vi "Write AI_AO_ALRState.vi"(0 "OPC UA server refnum in":T4, 1 "AI":T2, 2 "AI tags":string[](array[string]), 3 "AO":dbl[](array[numeric]), 4 "AO tags":string[](array[string]), 5 "error in (no error)":errorcluster, 6 "OPC UA AI list":string[](array[string]), 7 "ALR_State":T1, 9 "ALR tags":string[](array[string])) -> (14 "OPC UA server refnum out":T4, 19 "error out":errorcluster)   [LabVIEW 2019, in "OPC addons.lvlib"]
uses:
  OPC addons.lvlib
  <vilib>/OPCUA/controls/OPC UA Server Refnum.ctl
  Inputs/Ctl/AI short.ctl
  Inputs/Ctl/Parameter State.ctl
  Alarms/Ctl/ALRs_State.ctl
  <vilib>/OPCUA/controls/Write Status.ctl
  <vilib>/OPCUA/server/Write Variant.vi
  <vilib>/OPCUA/NI OPC UA Server.lvlib
  Alarms/Alarms.lvlib
  Inputs/Inputs.lvlib
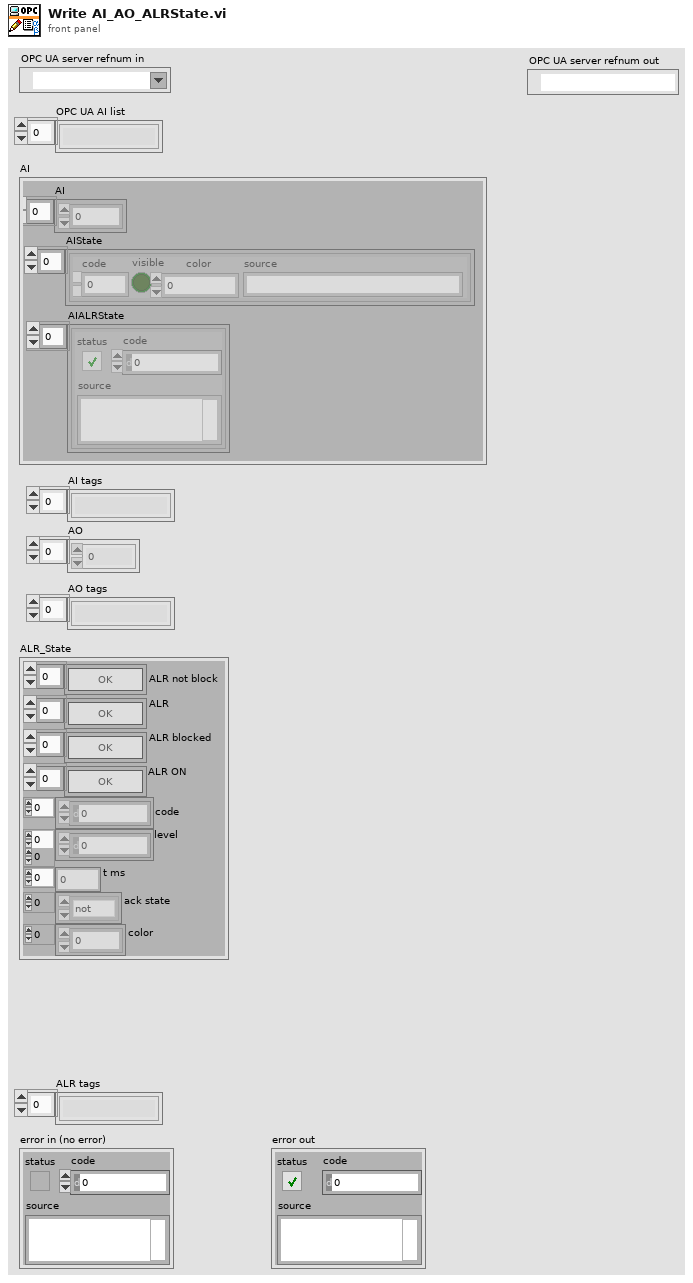
[diagram p1: front panel]
types:
  T1 = typedef "Alarms.lvlib/ALRs_State.ctl" = cluster{"ALR not block":bool[], "ALR":bool[], "ALR blocked":bool[], "ALR ON":bool[], "code":i32[], "level":i32[][], "t ms":u32[], "ack state":enum32{"not", "tripped", "reset", "ack"}[], "color":u32[]}
  T2 = typedef "Inputs.lvlib/AI short.ctl" = cluster{"AI":dbl[], "AIState":T3[], "AIALRState":errorcluster[]}
  T3 = typedef "Inputs.lvlib/Parameter State.ctl" = cluster{"code":i32, "visible":bool, "color":u32, "source":string}
  T4 = typedef "OPC UA Server Refnum.ctl" = refnum<k21>
  T5 = typedef "Write Status.ctl" = u32
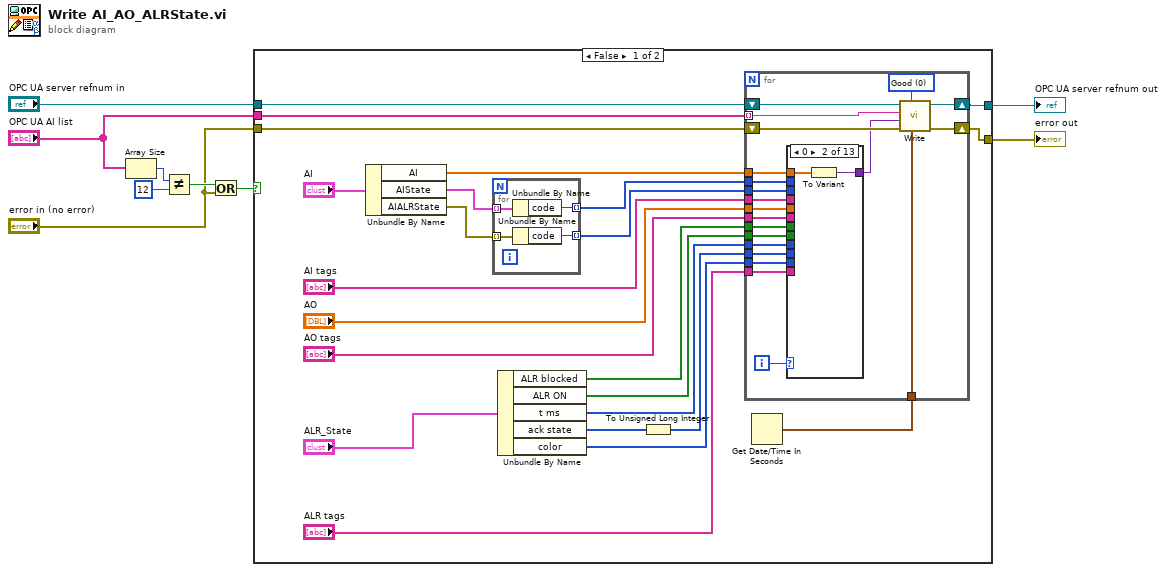
[diagram p0: block diagram]
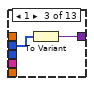
[diagram p3: hidden frame]
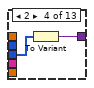
[diagram p4: hidden frame]
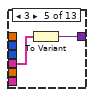
[diagram p5: hidden frame]
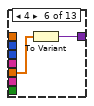
[diagram p6: hidden frame]
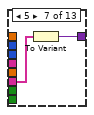
[diagram p7: hidden frame]
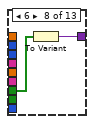
[diagram p8: hidden frame]
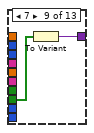
[diagram p9: hidden frame]
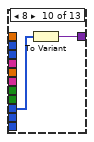
[diagram p10: hidden frame]
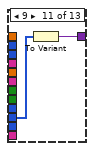
[diagram p11: hidden frame]
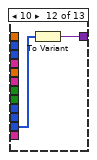
[diagram p12: hidden frame]
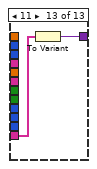
[diagram p13: hidden frame]
diagram:
  n1 = Array Size(array="OPC UA AI list") -> (size(s)=w5:i32)
  n2 = Not Equal?(x=w5, y=12) -> (x != y?=w3:bool)
  n3 = Or(x=w3, y="error in (no error)") -> (x .or. y?=w1:bool)
  n4 = case shown="False" w1 {
    tunnel: "OPC UA server refnum in" -> [w26 w83]
    tunnel: [w25 w83] -> w8
    tunnel: [w24 w82] -> w7
    tunnel: "OPC UA AI list" -> [w23 _]
    tunnel: "error in (no error)" -> [w22 w82]
    frame False {
      n5 = Unbundle By Name("AI") -> ("AI"=w30:dbl[], "AIState"=w31:T3[], "AIALRState"=w32:errorcluster[])
      n6 = for {
        tunnel: w31 -> [w81] mode=indexing
        tunnel: [w80] -> w21 mode=indexing
        tunnel: w32 -> [w79] mode=indexing
        tunnel: [w78] -> w20 mode=indexing
        n7 = Unbundle By Name(w81) -> ("code"=w80:i32)
        n8 = Unbundle By Name(w79) -> ("code"=w78:i32)
      }
      n9 = Unbundle By Name("ALR_State") -> ("ALR blocked"=w17:bool[], "ALR ON"=w18:bool[], "t ms"=w14:u32[], "ack state"=w13:enum32{"not", "tripped", "reset", "ack"}[], "color"=w11:u32[])
      n10 = To Unsigned Long Integer(number=w13) -> (unsigned 32bit integer=w12:u32[])
      n11 = Get Date/Time In Seconds() -> (seconds since 1Jan1904=w28:timestamp)
      n12 = for {
        tunnel: w28 -> [w39]
        tunnel: w30 -> [w53]
        tunnel: w21 -> [w51]
        tunnel: w23 -> [w37] mode=indexing
        tunnel: w20 -> [w50]
        tunnel: "AI tags" -> [w49]
        tunnel: "AO" -> [w48]
        tunnel: "AO tags" -> [w47]
        tunnel: w17 -> [w46]
        tunnel: w18 -> [w45]
        tunnel: w14 -> [w44]
        tunnel: w12 -> [w43]
        shift-right: [w36] -> w25
        shift-left: w26 -> [w41]
        shift-right: [w35] -> w24
        shift-left: w22 -> [w40]
        tunnel: w11 -> [w34]
        tunnel: "ALR tags" -> [w33]
        i -> [w52]
        w42 = T5 0 items=["Good"=0, "Uncertain"=1073741824, "Uncertain_InitialValue"=1083310080, "Uncertain_LastUsableValue"=1083179008, "Uncertain_SensorNotAccurate"=1083375616, "Uncertain_EngineeringUnitsExceeded"=1083441152, "Bad"=2147483648, "Bad_NoCommunication"=2150694912, "Bad_NotReadable"=2151284736, "Bad_NotWritable"=2151350272, "Bad_OutOfRange"=2151415808, "Bad_WaitingForInitialData"=2150760448] ("node status")
        n13 = case shown="0" w52 {
          tunnel: w53 -> [_ w55 _ _ _ _ _ _ _ _ _ _ _]
          tunnel: [_ w54 w57 w59 w61 w63 w65 w67 w69 w71 w73 w75 w77] -> w38
          tunnel: w51 -> [_ _ w56 _ _ _ _ _ _ _ _ _ _]
          tunnel: w50 -> [_ _ _ w58 _ _ _ _ _ _ _ _ _]
          tunnel: w49 -> [_ _ _ _ w60 _ _ _ _ _ _ _ _]
          tunnel: w48 -> [_ _ _ _ _ w62 _ _ _ _ _ _ _]
          tunnel: w47 -> [_ _ _ _ _ _ w64 _ _ _ _ _ _]
          tunnel: w46 -> [_ _ _ _ _ _ _ w66 _ _ _ _ _]
          tunnel: w45 -> [_ _ _ _ _ _ _ _ w68 _ _ _ _]
          tunnel: w44 -> [_ _ _ _ _ _ _ _ _ w70 _ _ _]
          tunnel: w43 -> [_ _ _ _ _ _ _ _ _ _ w72 _ _]
          tunnel: w34 -> [_ _ _ _ _ _ _ _ _ _ _ w74 _]
          tunnel: w33 -> [_ _ _ _ _ _ _ _ _ _ _ _ w76]
          frame -1, Default {
          }
          frame 0 {
            n14 = To Variant(anything=w55) -> (Variant=w54:variant)
          }
          frame 1 {
            n15 = To Variant(anything=w56) -> (Variant=w57:variant)
          }
          frame 2 {
            n16 = To Variant(anything=w58) -> (Variant=w59:variant)
          }
          frame 3 {
            n17 = To Variant(anything=w60) -> (Variant=w61:variant)
          }
          frame 4 {
            n18 = To Variant(anything=w62) -> (Variant=w63:variant)
          }
          frame 5 {
            n19 = To Variant(anything=w64) -> (Variant=w65:variant)
          }
          frame 6 {
            n20 = To Variant(anything=w66) -> (Variant=w67:variant)
          }
          frame 7 {
            n21 = To Variant(anything=w68) -> (Variant=w69:variant)
          }
          frame 8 {
            n22 = To Variant(anything=w70) -> (Variant=w71:variant)
          }
          frame 9 {
            n23 = To Variant(anything=w72) -> (Variant=w73:variant)
          }
          frame 10 {
            n24 = To Variant(anything=w74) -> (Variant=w75:variant)
          }
          frame 11 {
            n25 = To Variant(anything=w76) -> (Variant=w77:variant)
          }
        }
        n26 = call-poly <vilib>:"Write.vi"("timestamp (current time)"=w39, "node status"=w42, "error in (no error)"=w40, "value"=w38, "node ID"=w37, "OPC UA server refnum in"=w41) -> ("error out"=w35:errorcluster, "OPC UA server refnum out"=w36:T4)  [unwired: 3 in, 1 out]
      }
    }
    frame True {
    }
  }
  "OPC UA server refnum out" <- w8
  "error out" <- w7
